vi "robotModelTest.vi"(0 "Game in":refnum<class "Game.lvclass">, 1 "id":i32, 2 "Start":bool=TRUE, 3 "replace active":bool, 5 "V_sent":dbl, 7 "V_sample":dbl, 11 "error in (no error)":errorcluster, 13 "Samples":dbl, 14 "delta":dbl) -> (4 "Game out":refnum<class "Game.lvclass">, 6 "TestTeam":refnum<class "Ally.lvclass">, 8 "Replace":bool, 15 "error out":errorcluster)   [LabVIEW 2020, in "Game.lvclass"]
uses:
  Game.lvclass
  Controls/RobotModel.ctl
  Communication_class/Communication.lvclass
  Ally_class/Ally.lvclass
  C:/RoboIME/SSL_AI/Team_class/Team.lvclass
  Utilities_class/Utilities.lvclass
  Game.lvclass/Game.ctl
  Team_class/Team.lvclass/Team.ctl
  Robot_class/Robot.lvclass/Robot.ctl
  Object_class/Object.lvclass/Object.ctl
  Robot_class/Read est_v_tang.vi
  Robot_class/Write v_tang.vi
  Robot_class/Write v_norm.vi
  Robot_class/Write v_ang.vi
  Object_class/Read x.vi
  Object_class/Read y.vi
  <vilib>/Analysis/_algsub.llb/Real Vector Norm.vi
  Read TestTeam.vi
  Read AllyRef.vi
  Team_class/Read RobotRef.vi
  Robot_class/Read orientation.vi
  Team_class/Write RobotRef.vi
  Robot_class/Robot.lvclass
  C:/RoboIME/SSL_AI/Object_class/Object.lvclass
  <vilib>/Analysis/1siggen.llb/Ramp Pattern by Delta.vi
  <vilib>/Analysis/NI_AALPro.lvlib
  <vilib>/Analysis/NI_AALBase.lvlib
panel:
  out "Mean":T1[](array[typedef])
  out "Robot Model Array":T1[](array[typedef])
  in  "Communication in":refnum<class "Communication.lvclass">
  in  "Test Cluster":T1
  out "Waveform Chart":dbl(graph)
  out "Waveform Chart 2":dbl(graph)
  out "error out 2":errorcluster
  in  "error in (no error) 2":errorcluster
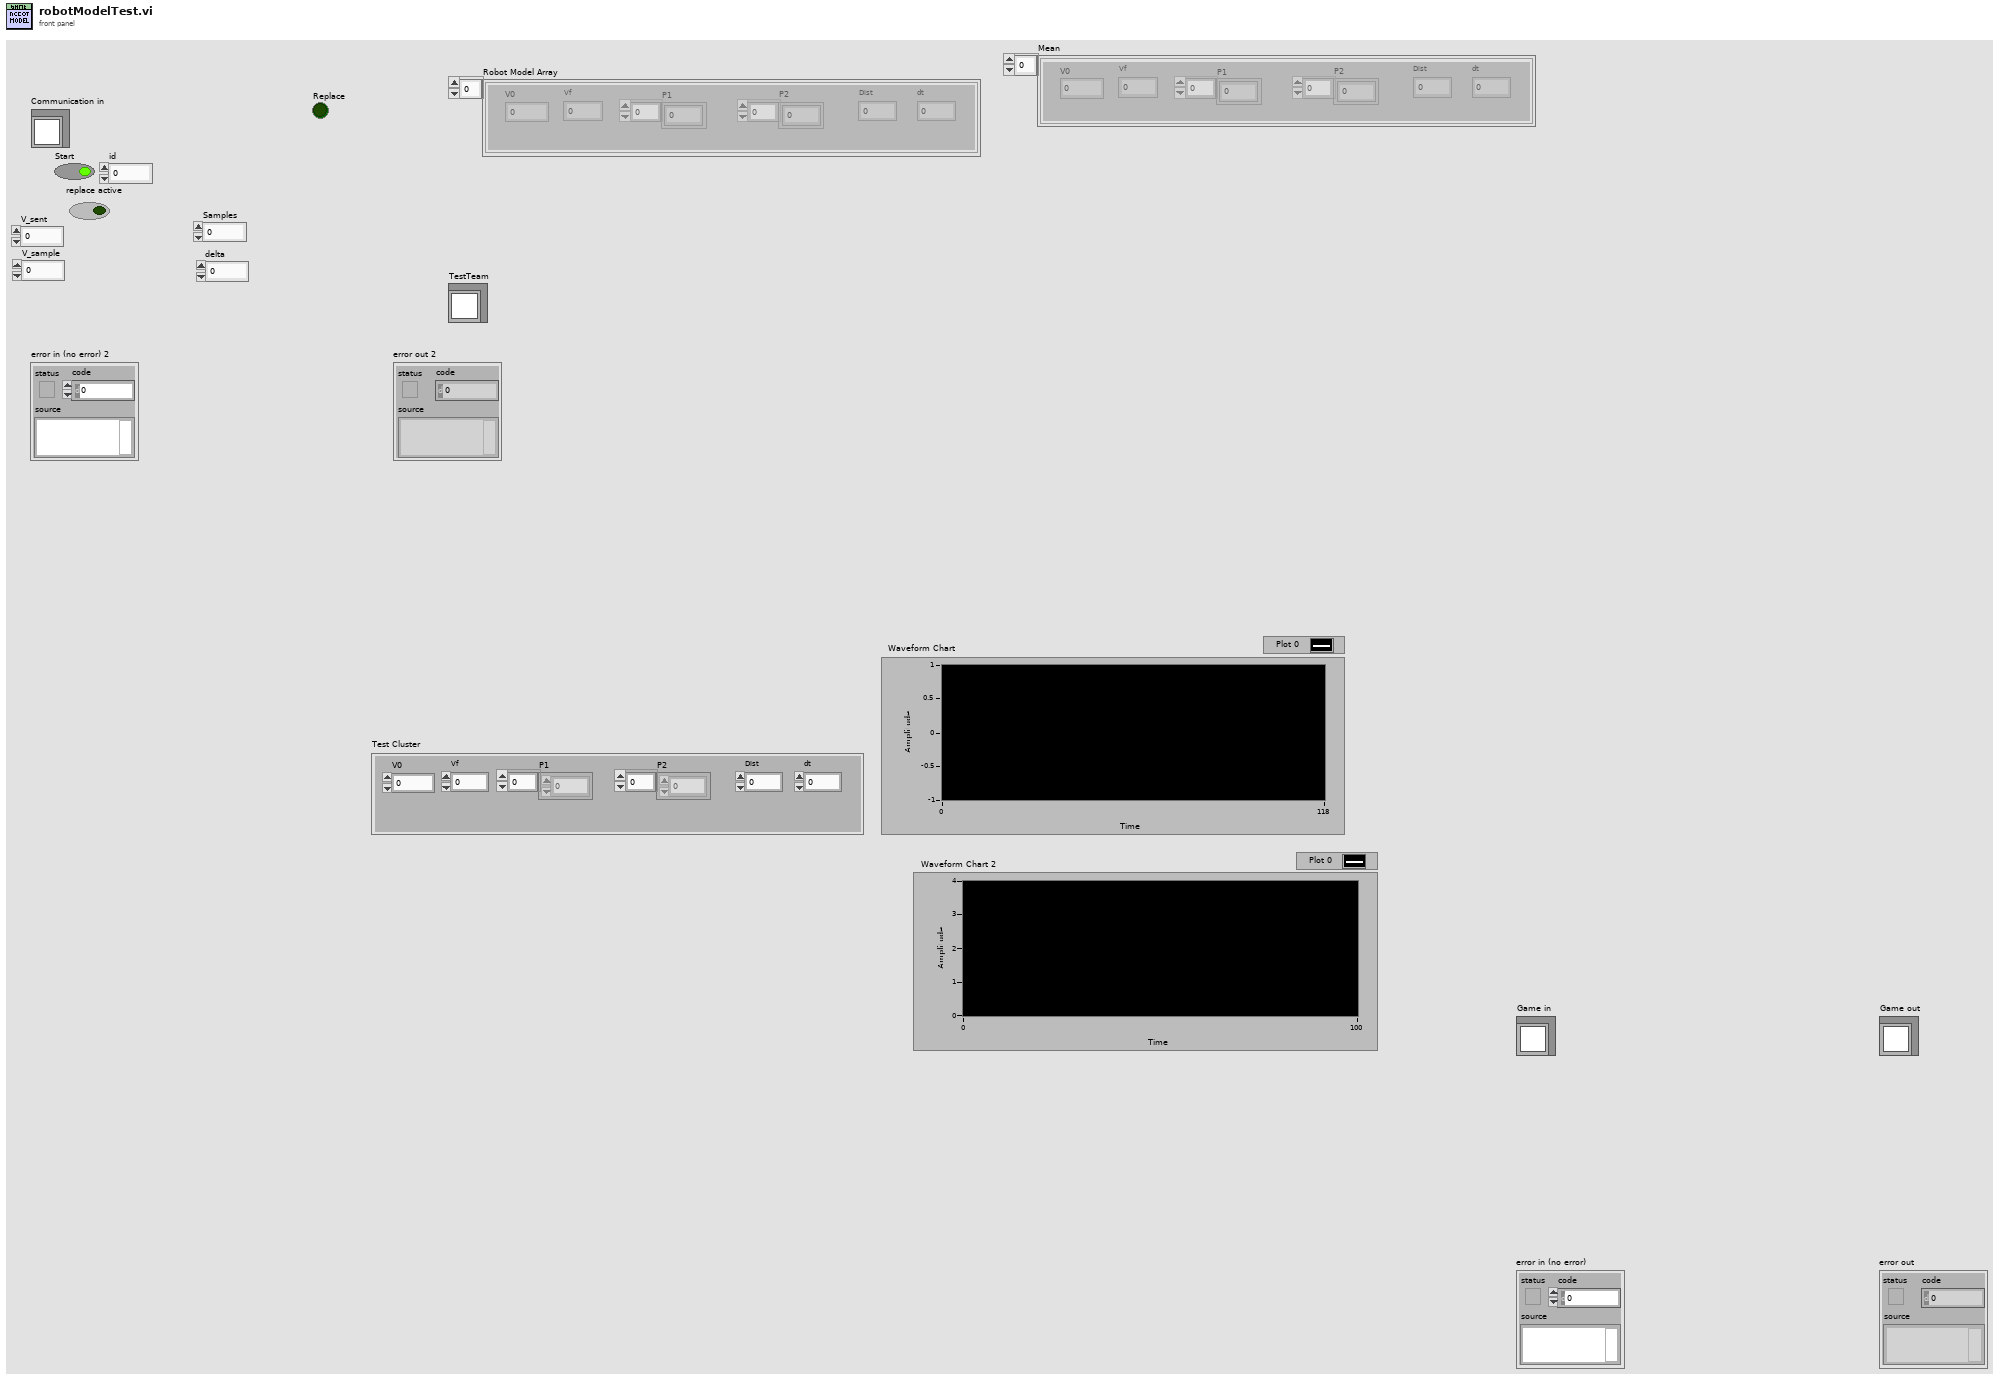
[diagram p1: front panel]
types:
  T1 = typedef "RobotModel.ctl" = cluster{"V0":dbl, "Vf":dbl, "Dist":dbl, "dt":dbl, "P1":dbl[], "P2":dbl[]}
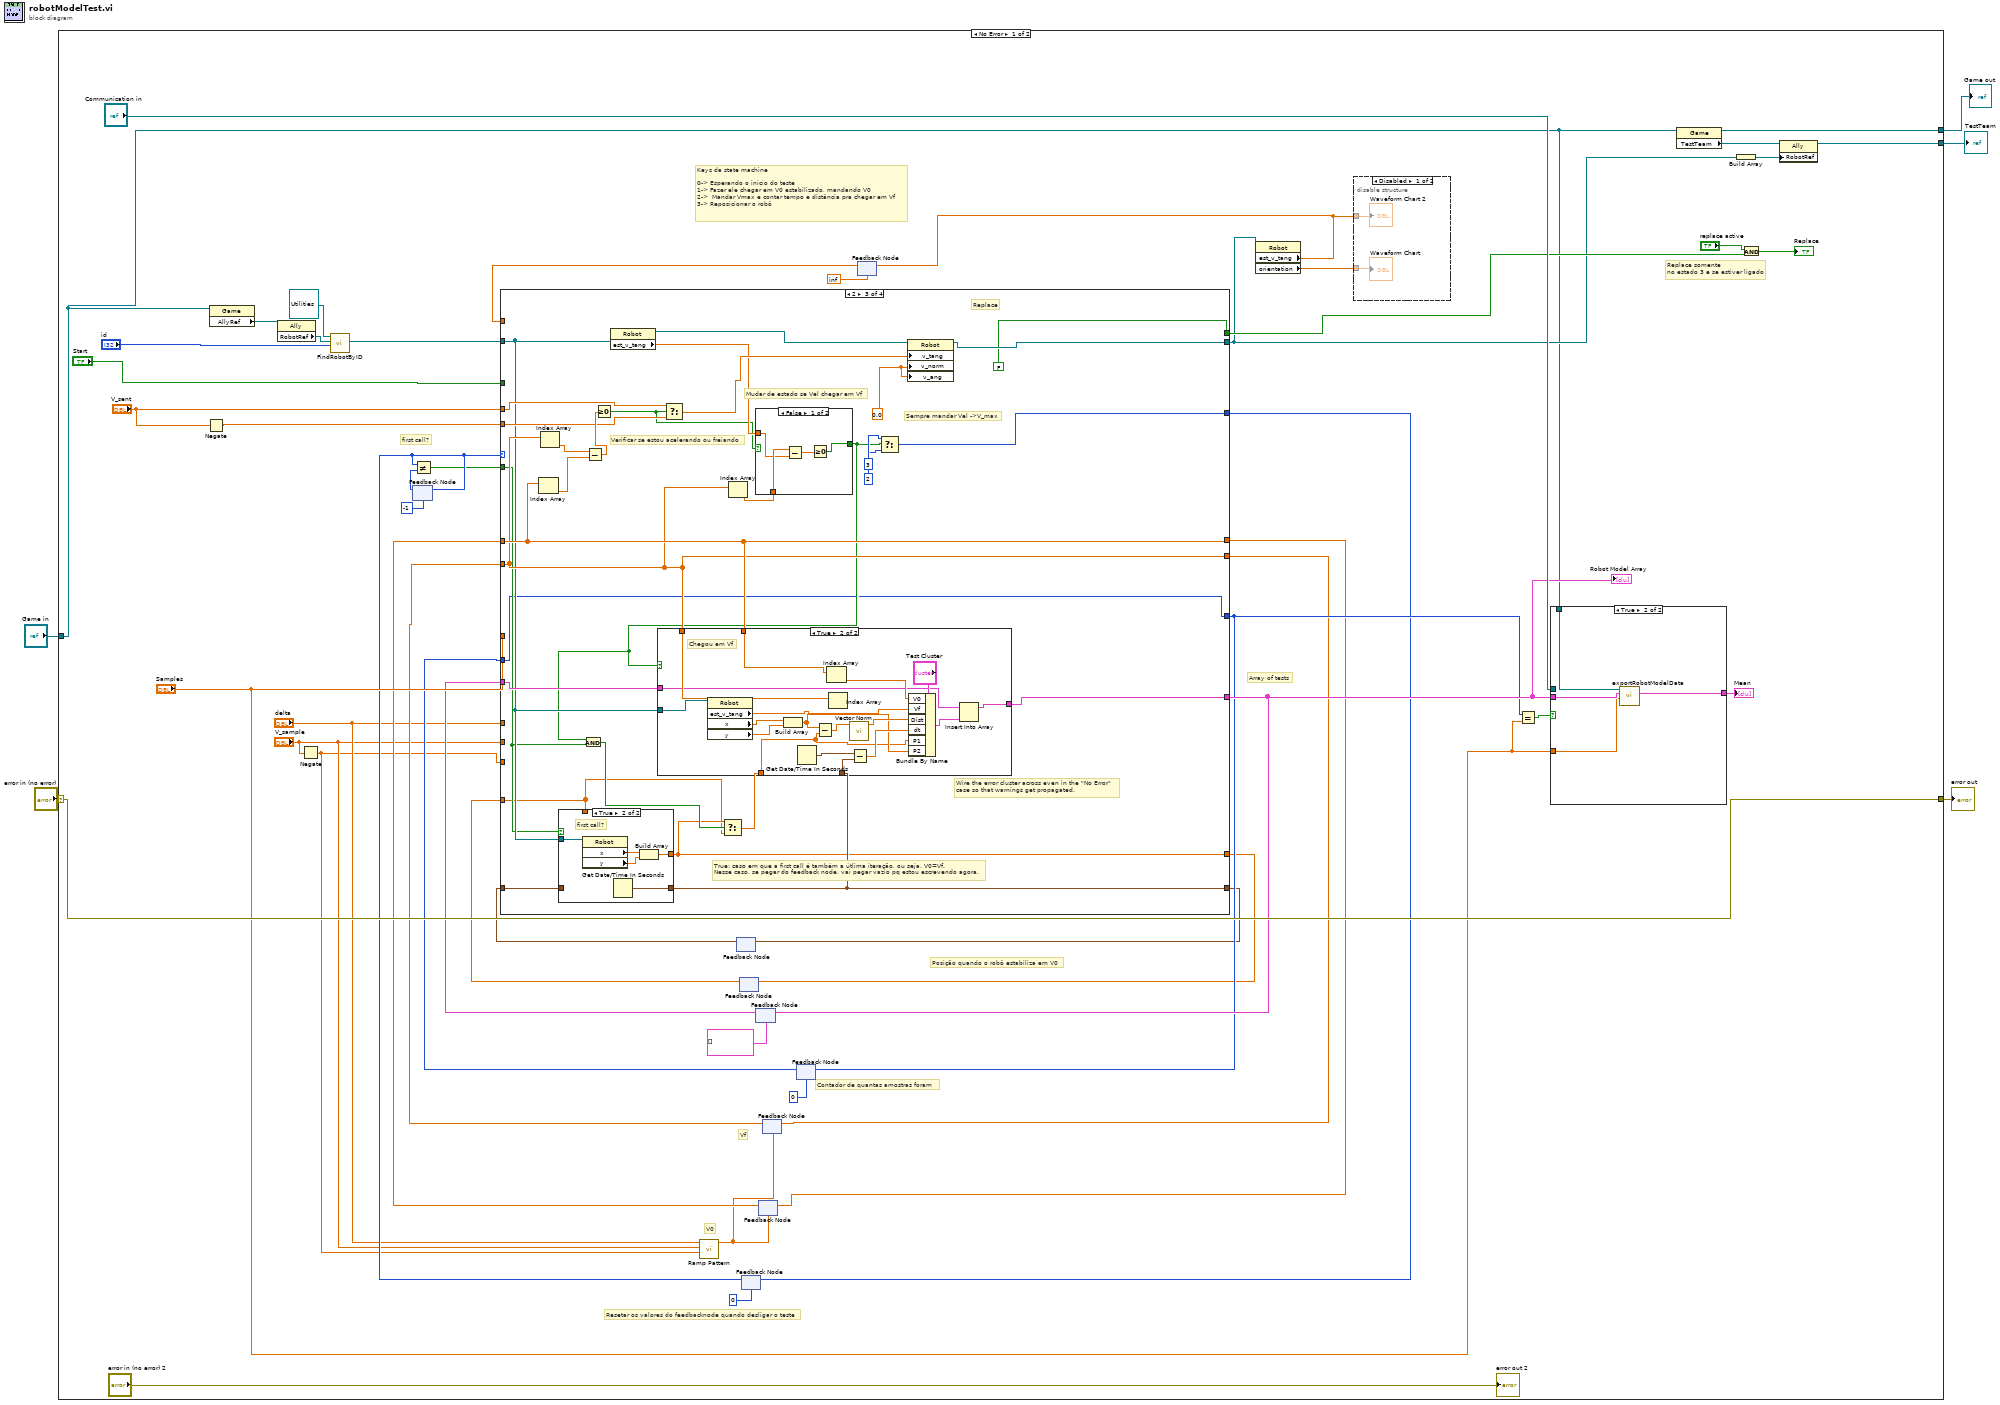
[diagram p0: block diagram]
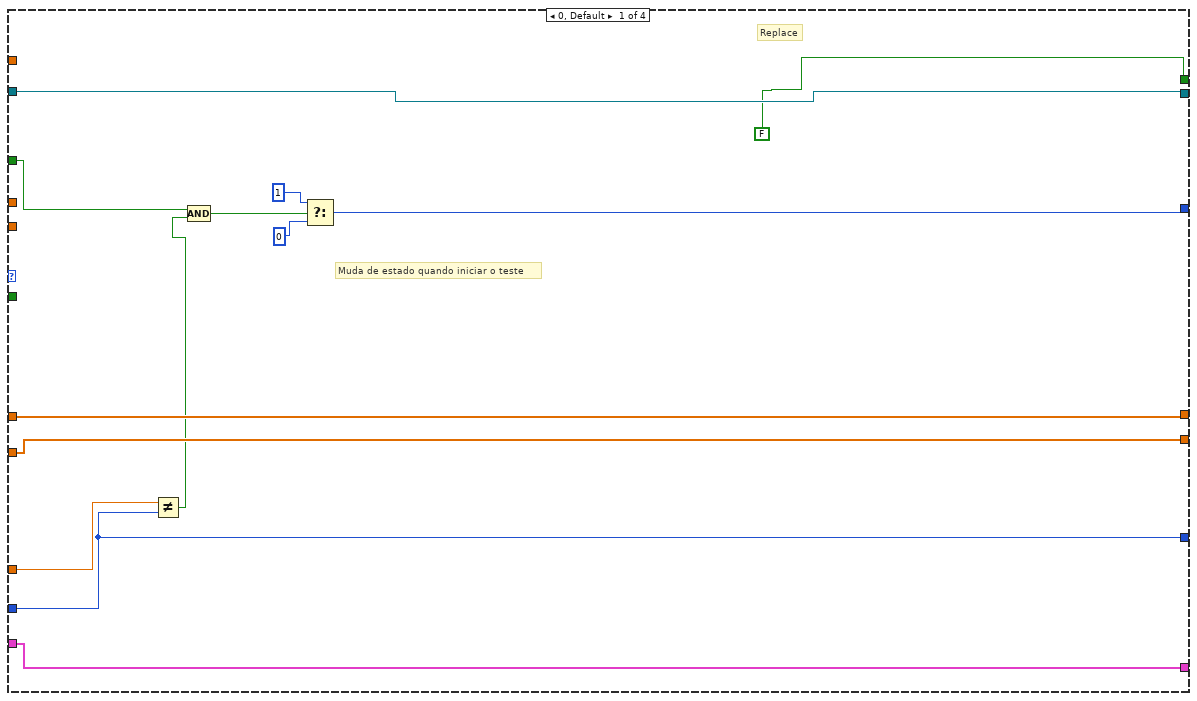
[diagram p3: hidden frame]
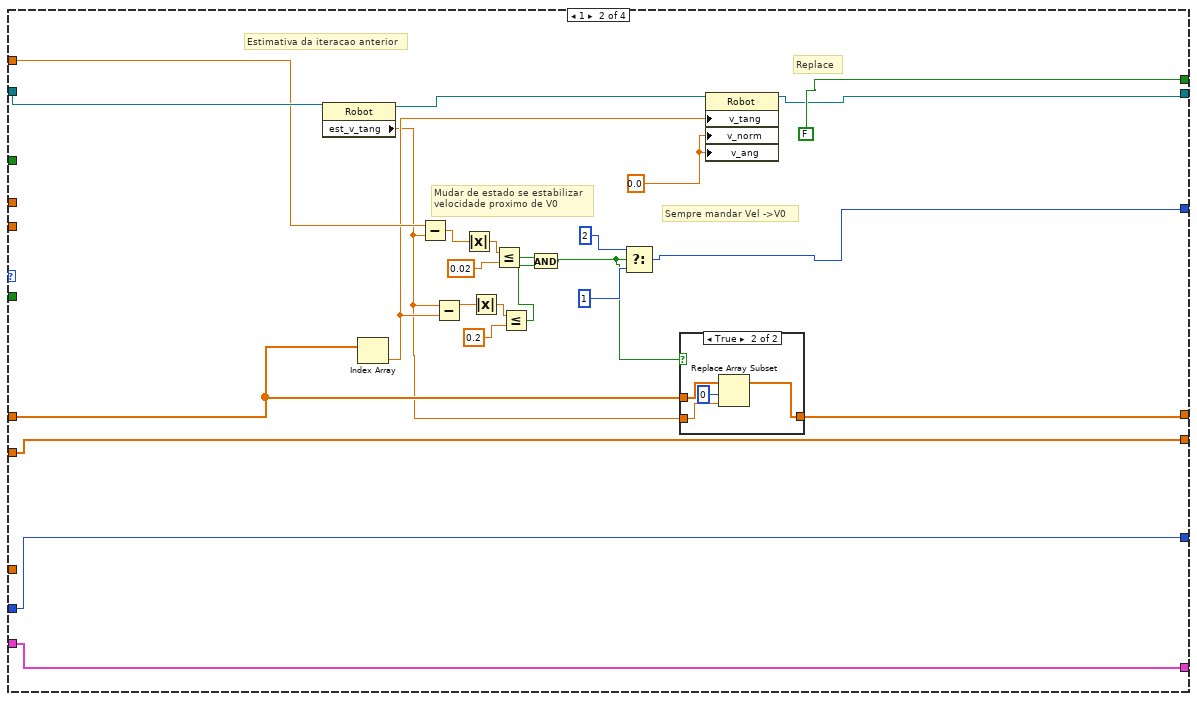
[diagram p4: hidden frame]
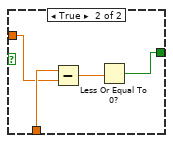
[diagram p6: hidden frame]
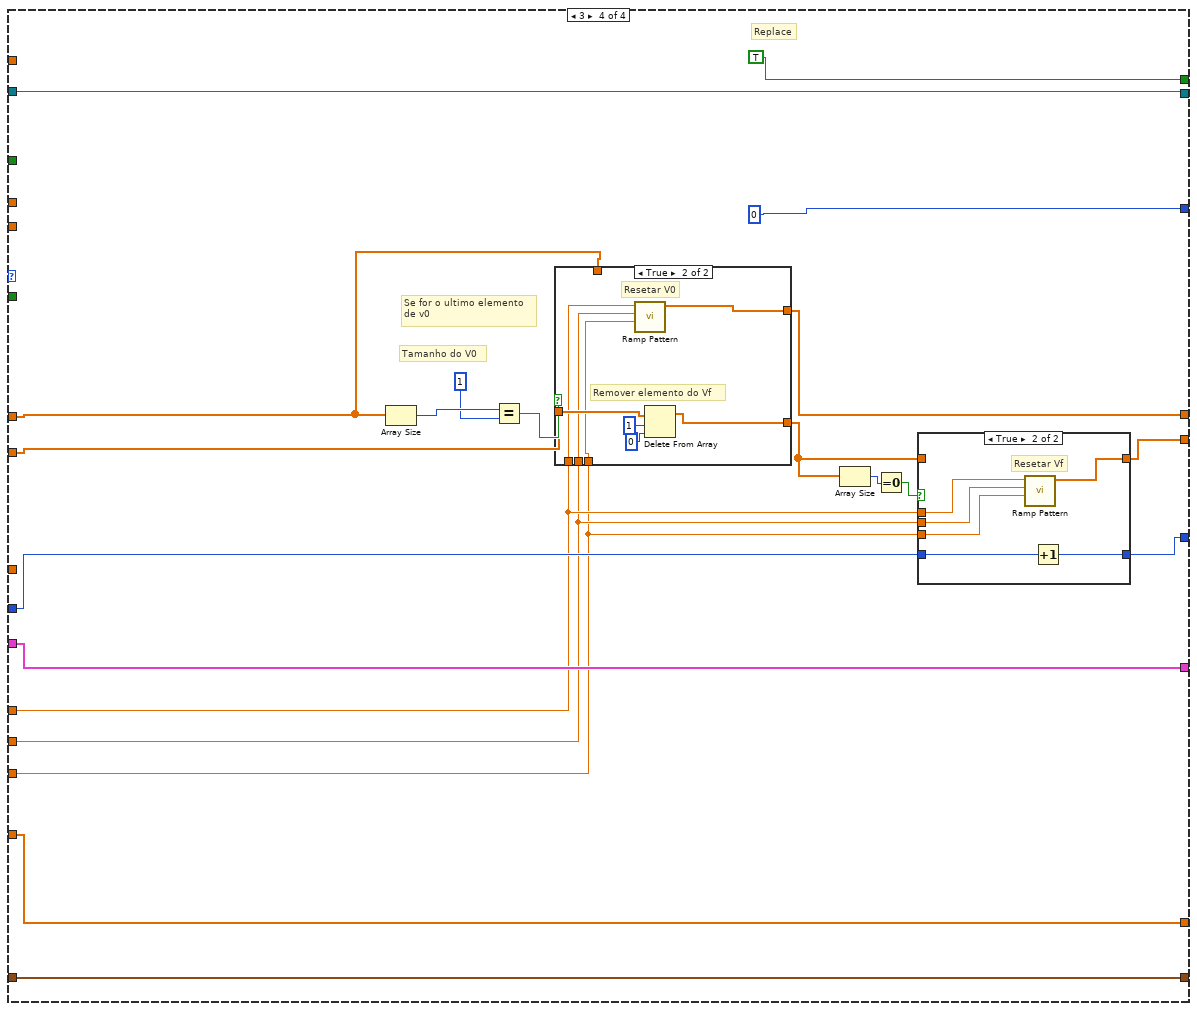
[diagram p9: hidden frame]
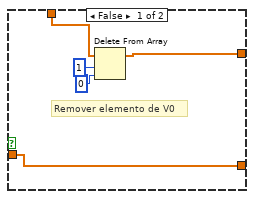
[diagram p11: hidden frame]
diagram:
  n1 = case shown="No Error" "error in (no error)" {
    selector: "error in (no error)" -> [w56 w212]
    tunnel: [w56 w212] -> w4
    tunnel: "Game in" -> [w16 _]
    tunnel: [w13 _] -> w2
    tunnel: [w14 _] -> w1
    frame No Error {
      # "Contador de quantas amostras foram"
      # "Posição quando o robô estabiliza em V0"
      # "Array of tests"
      # "first call?"
      # "Resetar os valores do feedbacknode quando desligar o teste"
      # "Vf"
      # "V0"
      # "Keys da state machine\n\n0-> Esperando o inicio do teste\n1-> Fazer ele chegar em V0 estabilizado, mandando V0\n2->  Mandar Vmax e contar tempo e distância pra chegar em Vf \n3-> Reposicionar o robô"
      # "Replace somente\nno estado 3 e se estiver ligado"
      # "Wire the error cluster across even in the \"No Error\"\ncase so that warnings get propagated."
      n2 = Negate(x="V_sent") -> (-x=w8:dbl)
      n3 = property class="Game"(reference=w16) -> ("AllyRef"=w42:refnum<class "Ally.lvclass">)  [unwired: 1 in, 2 out]
      n4 = property class="Ally"(reference=w42) -> ("RobotRef"=w41:refnum<class "Robot.lvclass">[])  [unwired: 1 in, 2 out]
      n5 = Negate(x="V_sample") -> (-x=w6:dbl)
      n6 = call-dynamic "FindRobotByID.vi"("id"="id", "RobotRef"=w41, "Utilities in"=refnum<class "Utilities.lvclass"> refnum) -> ("Robot"=w39:refnum<class "Robot.lvclass">)  [unwired: 5 in, 3 out]
      n7 = feedback #1(-1) -> (w29:i32)
      n8 = call-poly <vilib>:"Ramp Pattern.vi"("start"=w6, "end"="V_sample", "delta"="delta") -> ("Ramp Pattern"=w11:dbl[])  [unwired: 6 in, 2 out]
      n9 = feedback #2() -> (w34:timestamp)  [unwired: 1 in]
      n10 = feedback #3() -> (w33:dbl[])  [unwired: 1 in]
      n11 = feedback #4(0) -> (w26:i32)
      n12 = feedback-in #1(w26) -> ()
      n13 = Not Equal?(x=w26, y=w29) -> (x != y?=w25:bool)
      n14 = feedback #5(T1[] [] ("Array")) -> (w32:T1[])
      n15 = feedback #6(w11) -> (w30:dbl[])
      n16 = feedback #7(w11) -> (w31:dbl[])
      n17 = feedback #8(0) -> (w21:i32)
      n18 = feedback #9(inf) -> (w24:dbl)
      n19 = case shown="2" w26 {
        tunnel: "Start" -> [w65 _ _ _]
        tunnel: [w69 w77 w126 0] -> w43
        tunnel: w39 -> [w67 w88 w114 w180]
        tunnel: w30 -> [w68 w76 w118 w179]
        tunnel: w31 -> [w66 w90 w117 w177]
        tunnel: "V_sent" -> [_ _ w124 _]
        tunnel: w8 -> [_ _ w123 _]
        tunnel: [w67 w86 w131 w180] -> w19
        tunnel: [w68 w74 w118 w182] -> w37
        tunnel: [w66 w90 w117 w171] -> w38
        tunnel: [FALSE FALSE FALSE TRUE] -> w51
        tunnel: [_ _ w115 w175] -> w36
        tunnel: [_ _ w109 w178] -> w35
        tunnel: w34 -> [_ _ w119 w175]
        tunnel: w33 -> [_ _ w108 w178]
        tunnel: [w62 w87 w113 w176] -> w48
        tunnel: w32 -> [w62 w87 w116 w176]
        tunnel: w25 -> [_ _ w112 _]
        tunnel: w24 -> [_ w84 _ _]
        tunnel: "Samples" -> [w60 _ _ _]
        tunnel: [w61 w72 w104 w170] -> w46
        tunnel: w21 -> [w61 w72 w104 w169]
        tunnel: "delta" -> [_ _ _ w168]
        tunnel: "V_sample" -> [_ _ _ w167]
        tunnel: w6 -> [_ _ _ w166]
        frame 0, Default {
          # "Replace"
          # "Muda de estado quando iniciar o teste"
          n20 = Not Equal?(x=w60, y=w61) -> (x != y?=w59:bool)
          n21 = Compound Arithmetic op=AND(w65, w59) -> (w64:bool)
          n22 = Select(t=1, s=w64, f=0) -> (s? t:f=w69:i32)
        }
        frame 1 {
          w96 = 0.0 ("v_norm")
          # "Estimativa da iteracao anterior"
          # "Replace"
          # "Mudar de estado se estabilizar\nvelocidade proximo de V0"
          # "Sempre mandar Vel ->V0"
          n23 = property class="Robot"(reference=w88) -> (reference out=w95:refnum<class "Robot.lvclass">, "est_v_tang"=w73:dbl)  [unwired: 1 in, 1 out]
          n24 = Index Array(array=w76) -> (element=w80:dbl)  [unwired: 1 in]
          n25 = Subtract(x=w84, y=w73) -> (x-y=w85:dbl)
          n26 = Subtract(x=w73, y=w80) -> (x-y=w83:dbl)
          n27 = Absolute Value(x=w85) -> (abs(x)=w94:dbl)
          n28 = Absolute Value(x=w83) -> (abs(x)=w81:dbl)
          n29 = Less Or Equal?(x=w94, y=0.02) -> (x <= y?=w79:bool)
          n30 = Less Or Equal?(x=w81, y=0.2) -> (x <= y?=w78:bool)
          n31 = And(x=w79, y=w78) -> (x .and. y?=w75:bool)
          n32 = Select(t=2, s=w75, f=1) -> (s? t:f=w77:i32)
          n33 = case shown="True" w75 {
            tunnel: w76 -> [w97 w101]
            tunnel: [w97 w98] -> w74
            tunnel: w73 -> [_ w100]
            frame False {
            }
            frame True {
              n34 = Replace Array Subset(array=w101, new element=w100, index=0) -> (w98:dbl[])
            }
          }
          n35 = property class="Robot"(reference=w95, "v_tang"=w80, "v_norm"=w96, "v_ang"=w96) -> (reference out=w86:refnum<class "Robot.lvclass">)  [unwired: 1 in, 1 out]
        }
        frame 2 {
          w130 = 0.0 ("v_norm")
          # "True: caso em que a first call é também a útlima iteração, ou seja, V0=Vf.\nNesse caso, se pegar do feedback node, vai pegar vazio pq estou escrevendo agora."
          # "Replace"
          # "Verificar se estou acelerando ou freiando"
          # "Mudar de estado se Vel chegar em Vf"
          # "Sempre mandar Vel ->V_max"
          n36 = Index Array(array=w118) -> (element=w102:dbl)  [unwired: 1 in]
          n37 = Index Array(array=w117) -> (element=w103:dbl)  [unwired: 1 in]
          n38 = case shown="True" w112 {
            tunnel: [w160 w165] -> w115
            tunnel: w119 -> [w160 _]
            tunnel: w114 -> [_ w164]
            tunnel: [w159 w161] -> w109
            tunnel: w108 -> [w159 _]
            frame False {
            }
            frame True {
              # "first call?"
              n39 = property class="Robot"(reference=w164) -> ("x"=w163:dbl, "y"=w162:dbl)  [unwired: 1 in, 2 out]
              n40 = Get Date/Time In Seconds() -> (seconds since 1Jan1904=w165:timestamp)
              n41 = Build Array(w163, w162) -> (w161:dbl[])
            }
          }
          n42 = Subtract(x=w103, y=w102) -> (x-y=w125:dbl)
          n43 = Greater Or Equal To 0?(x=w125) -> (x >= 0?=w105:bool)
          n44 = property class="Robot"(reference=w114) -> (reference out=w129:refnum<class "Robot.lvclass">, "est_v_tang"=w106:dbl)  [unwired: 1 in, 1 out]
          n45 = Select(t=w124, s=w105, f=w123) -> (s? t:f=w122:dbl)
          n46 = Index Array(array=w117) -> (element=w120:dbl)  [unwired: 1 in]
          n47 = case shown="False" w105 {
            tunnel: w120 -> [w135 w139]
            tunnel: [w132 w136] -> w111
            tunnel: w106 -> [w134 w138]
            frame False {
              n48 = Subtract(x=w135, y=w134) -> (x-y=w133:dbl)
              n49 = Greater Or Equal To 0?(x=w133) -> (x >= 0?=w132:bool)
            }
            frame True {
              n50 = Subtract(x=w139, y=w138) -> (x-y=w137:dbl)
              n51 = Less Or Equal To 0?(x=w137) -> (x <= 0?=w136:bool)
            }
          }
          n52 = And(x=w111, y=w112) -> (x .and. y?=w110:bool)
          n53 = Select(t=w109, s=w110, f=w108) -> (s? t:f=w107:dbl[])
          n54 = case shown="True" w111 {
            tunnel: w118 -> [_ w152]
            tunnel: w117 -> [_ w151]
            tunnel: w114 -> [_ w150]
            tunnel: w116 -> [w140 w145]
            tunnel: [w140 w143] -> w113
            tunnel: w115 -> [_ w148]
            tunnel: w107 -> [_ w142]
            frame False {
            }
            frame True {
              # "Chegou em Vf"
              n55 = property class="Robot"(reference=w150) -> ("est_v_tang"=w141:dbl, "x"=w158:dbl, "y"=w157:dbl)  [unwired: 1 in, 2 out]
              n56 = Build Array(w158, w157) -> (w146:dbl[])
              n57 = Get Date/Time In Seconds() -> (seconds since 1Jan1904=w149:timestamp)
              n58 = Subtract(x=w146, y=w142) -> (x-y=w155:dbl[])
              n59 = Index Array(array=w152) -> (element=w153:dbl)  [unwired: 1 in]
              n60 = Index Array(array=w151) -> ()  [unwired: 1 in, 1 out]
              n61 = call-poly <vilib>:"Vector Norm.vi"("Input Vector"=w155) -> ("norm"=w154:dbl)  [unwired: 9 in, 1 out]
              n62 = Subtract(x=w149, y=w148) -> (x-y=w147:dbl)
              n63 = Bundle By Name(cluster="Test Cluster", "V0"=w153, "Vf"=w141, "Dist"=w154, "dt"=w147, "P1"=w142, "P2"=w146) -> (w144:T1)
              n64 = Insert Into Array(array=w145, new element=w144) -> (w143:T1[])  [unwired: 1 in]
            }
          }
          n65 = Select(t=3, s=w111, f=2) -> (s? t:f=w126:i32)
          n66 = property class="Robot"(reference=w129, "v_tang"=w122, "v_norm"=w130, "v_ang"=w130) -> (reference out=w131:refnum<class "Robot.lvclass">)  [unwired: 1 in, 1 out]
        }
        frame 3 {
          # "Se for o ultimo elemento\nde v0"
          # "Replace"
          # "Tamanho do V0"
          n67 = Array Size(array=w179) -> (size(s)=w185:i32)
          n68 = Equal?(x=w185, y=1) -> (x = y?=w183:bool)
          n69 = case shown="True" w183 {
            tunnel: [w196 w207] -> w182
            tunnel: w179 -> [w199 _]
            tunnel: w177 -> [w195 w206]
            tunnel: [w195 w203] -> w172
            tunnel: w168 -> [_ w202]
            tunnel: w167 -> [_ w201]
            tunnel: w166 -> [_ w200]
            frame False {
              # "Remover elemento de V0"
              n70 = Delete From Array(array=w199, length=1, index=0) -> (array with subset deleted=w196:dbl[])  [unwired: 1 out]
            }
            frame True {
              # "Remover elemento do Vf"
              # "Resetar V0"
              n71 = call-poly <vilib>:"Ramp Pattern.vi"("start"=w200, "end"=w201, "delta"=w202) -> ("Ramp Pattern"=w207:dbl[])  [unwired: 6 in, 2 out]
              n72 = Delete From Array(array=w206, length=1, index=0) -> (array with subset deleted=w203:dbl[])  [unwired: 1 out]
            }
          }
          n73 = Array Size(array=w172) -> (size(s)=w174:i32)
          n74 = Equal To 0?(x=w174) -> (x = 0?=w173:bool)
          n75 = case shown="True" w173 {
            tunnel: w172 -> [w188 _]
            tunnel: [w188 w194] -> w171
            tunnel: [w187 w193] -> w170
            tunnel: w169 -> [w187 w192]
            tunnel: w168 -> [_ w191]
            tunnel: w167 -> [_ w190]
            tunnel: w166 -> [_ w189]
            frame False {
            }
            frame True {
              # "Resetar Vf"
              n76 = call-poly <vilib>:"Ramp Pattern.vi"("start"=w189, "end"=w190, "delta"=w191) -> ("Ramp Pattern"=w194:dbl[])  [unwired: 6 in, 2 out]
              n77 = Increment(x=w192) -> (x+1=w193:i32)
            }
          }
        }
      }
      "Robot Model Array" <- w48
      n78 = feedback-in #2(w36) -> ()
      n79 = feedback-in #3(w35) -> ()
      n80 = feedback-in #4(w43) -> ()
      n81 = feedback-in #5(w48) -> ()
      n82 = feedback-in #6(w37) -> ()
      n83 = feedback-in #7(w38) -> ()
      n84 = feedback-in #8(w46) -> ()
      n85 = property class="Robot"(reference=w19) -> ("est_v_tang"=w20:dbl, "orientation"=w12:dbl)  [unwired: 1 in, 2 out]
      n86 = feedback-in #9(w20) -> ()
      n87 = disable-structure shown="Disabled" {
        disable-tunnel: w20 -> [w58 _]
        disable-tunnel: w12 -> [w57 _]
        frame Disabled {
          "Waveform Chart" <- w57
          "Waveform Chart 2" <- w58
        }
        frame Enabled {
        }
      }
      n88 = Equal?(x=w46, y="Samples") -> (x = y?=w45:bool)
      n89 = case shown="True" w45 {
        tunnel: "Samples" -> [_ w209]
        tunnel: "Communication in" -> [_ _]
        tunnel: w48 -> [_ w211]
        tunnel: w16 -> [_ w210]
        tunnel: [_ w208] -> w15
        frame False {
        }
        frame True {
          n90 = call "exportRobotModelData.vi"("Samples"=w209, "Robot Model Array"=w211, "Game in"=w210) -> ("Mean"=w208:T1[])  [unwired: 6 in, 2 out]
        }
      }
      "Mean" <- w15
      n91 = property class="Game"(reference=w16) -> (reference out=w13:refnum<class "Game.lvclass">, "TestTeam"=w17:refnum<class "Ally.lvclass">)  [unwired: 1 in, 1 out]
      n92 = Build Array(w19) -> (w18:refnum<class "Robot.lvclass">[])
      n93 = And(x="replace active", y=w51) -> (x .and. y?=→"Replace":bool)
      n94 = property class="Ally"(reference=w17, "RobotRef"=w18) -> (reference out=w14:refnum<class "Ally.lvclass">)  [unwired: 1 in, 1 out]
      "error out 2" <- "error in (no error) 2"
    }
    frame Error {
    }
  }
  "error out" <- w4
  "Game out" <- w2
  "TestTeam" <- w1
